vi "opencvSelectCandidateNeurons5Planes.vi"(0 "ArrB0":sgl[](array[numeric]), 1 "ArrB1":sgl[](array[numeric]), 2 "ArrB2":sgl[](array[numeric]), 3 "ArrB3":sgl[](array[numeric]), 4 "ArrB4":sgl[](array[numeric]), 5 "NeuronXYin":u16[](array[numeric]), 6 "sizeBx":i32, 7 "NeuronNin":u16, 8 "sizeBy":i32, 9 "NeuronXYout":u16[](array[numeric]), 11 "NeuronNout":u16) -> (14 "ArrB1 out":sgl[](array[numeric]), 15 "ArrB2 out":sgl[](array[numeric]), 16 "ArrB3 out":sgl[](array[numeric]), 17 "ArrB4 out":sgl[](array[numeric]), 18 "NeuronXYout out":u16[](array[numeric]), 19 "NeuronNout out":u16)   [LabVIEW 2017]
uses:
  dll/wormUtilities/x64/Release/wormUtilities.dll
panel:
  out "NeuronNin out":u16
  out "NeuronXYin out":u16[](array[numeric])
  out "sizeBy out":i32
  out "sizeBx out":i32
  out "ArrB0 out":sgl[](array[numeric])
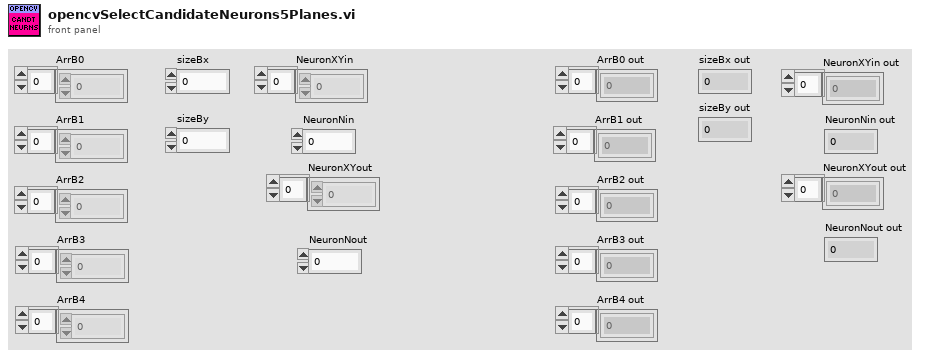
[diagram p1: front panel]
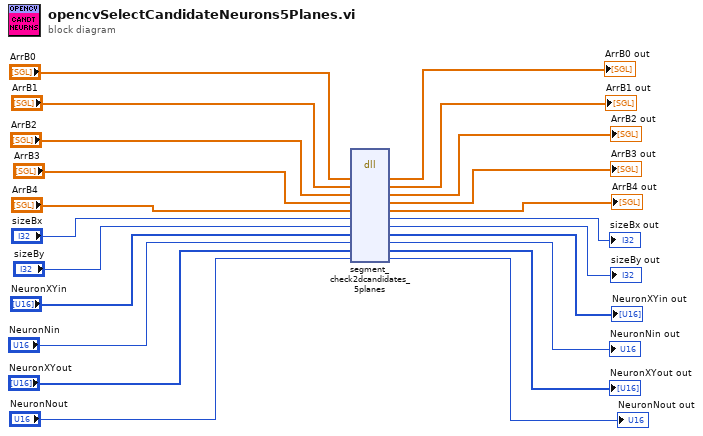
[diagram p0: block diagram]
diagram:
  n1 = dll-call lib="C:/Users/francesco/dev/pump-probe/dll/wormUtilities/x64/Release/wormUtilities.dll" fn="segment_check2dcandidates_5planes"("ArrB0"="ArrB0", "ArrB1"="ArrB1", "ArrB2"="ArrB2", "ArrB3"="ArrB3", "ArrB4"="ArrB4", "sizeBx"="sizeBx", "sizeBy"="sizeBy", "NeuronXYin"="NeuronXYin", "NeuronNin"="NeuronNin", "NeuronXYout"="NeuronXYout", "NeuronNout"="NeuronNout") -> ("ArrB0"=→"ArrB0 out":sgl[], "ArrB1"=→"ArrB1 out":sgl[], "ArrB2"=→"ArrB2 out":sgl[], "ArrB3"=→"ArrB3 out":sgl[], "ArrB4"=→"ArrB4 out":sgl[], "sizeBx"=→"sizeBx out":i32, "sizeBy"=→"sizeBy out":i32, "NeuronXYin"=→"NeuronXYin out":u16[], "NeuronNin"=→"NeuronNin out":u16, "NeuronXYout"=→"NeuronXYout out":u16[], "NeuronNout"=→"NeuronNout out":u16)  [unwired: 4 in, 2 out]
